vi "Cal RHS (Numeric).vi"(8 "error in (no error)":errorcluster, 10 "RHS in":variant, 11 "Domain in":refnum<class "NI_Domain.lvclass">) -> (0 "error out":errorcluster, 2 "RHS out":variant, 3 "Domain out":refnum<class "NI_Domain.lvclass">)   [LabVIEW 2020, in "NI_PDE.lvlib" / "NI_Domain.lvclass"]
uses:
  <vilib>/gmath/pde.llb/DomainClass/NI_Domain.lvclass
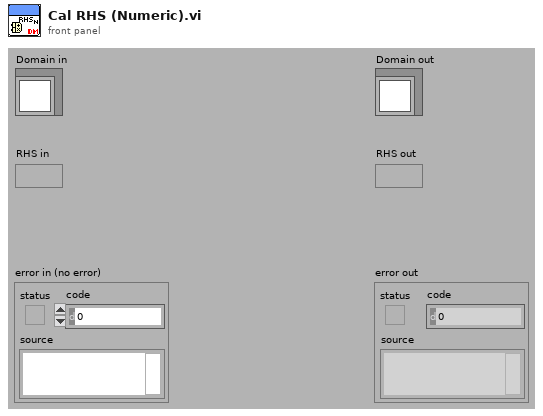
[diagram p1: front panel]
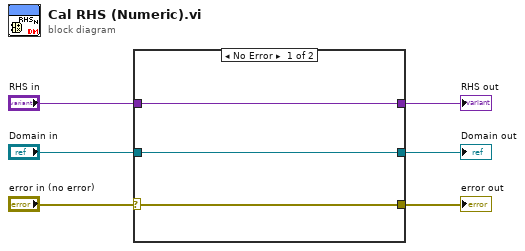
[diagram p0: block diagram]
diagram:
  n1 = case shown="No Error" "error in (no error)" {
    selector: "error in (no error)" -> [w8 w12]
    tunnel: "Domain in" -> [w9 w11]
    tunnel: [w9 w11] -> w6
    tunnel: [w8 w12] -> w5
    tunnel: [w7 w10] -> w2
    tunnel: "RHS in" -> [w7 w10]
    frame No Error {
    }
    frame Error {
    }
  }
  "Domain out" <- w6
  "error out" <- w5
  "RHS out" <- w2
